vi "test Convert Endpoint to UI Element.vi"(8 "error in (no error)":errorcluster, 11 "TestCase in":refnum<class "SLSC Switch Unit Tests.lvclass">) -> (0 "error out":errorcluster, 3 "TestCase out":refnum<class "SLSC Switch Unit Tests.lvclass">)   [LabVIEW 2017, in "SLSC Switch Unit Tests.lvclass"]
uses:
  SLSC Switch Unit Tests.lvclass
  Shared/Endpoint Configuration Enum.ctl
  System Explorer/Channel Type.ctl
  Shared/Endpoint Configuration Cluster.ctl
  <vilib>/addons/_JKI Toolkits/VI Tester/TestCase.llb/TestCase.lvclass
  System Explorer/SLSC Switch System Explorer.lvlib
  Shared/SLSC Switch Shared.lvlib
  C:/Program Files (x86)/National Instruments/LabVIEW 2017/vi.lib/addons/_JKI Toolkits/VI Tester/TestCase.llb/TestCase.lvclass
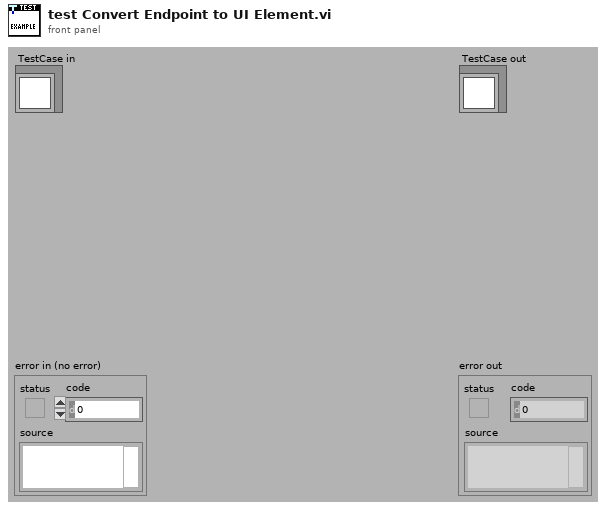
[diagram p1: front panel]
types:
  T1 = typedef "SLSC Switch Shared.lvlib/Endpoint Configuration Enum.ctl" = enum16{"Load", "Source", "Configuration"}
  T2 = typedef "SLSC Switch System Explorer.lvlib/Channel Type.ctl" = enum16{"Load (Default)", "Source", "Configuration"}
  T3 = cluster{"Configuration":T1, "Configuration 2":T2}[]
  T4 = typedef "SLSC Switch Shared.lvlib/Endpoint Configuration Cluster.ctl" = cluster{"Endpoint":string, "Configuration":T1}
  T5 = typedef "SLSC Switch System Explorer.lvlib/Channel.ctl" = cluster{"Endpoint":string, "Configuration":T2}
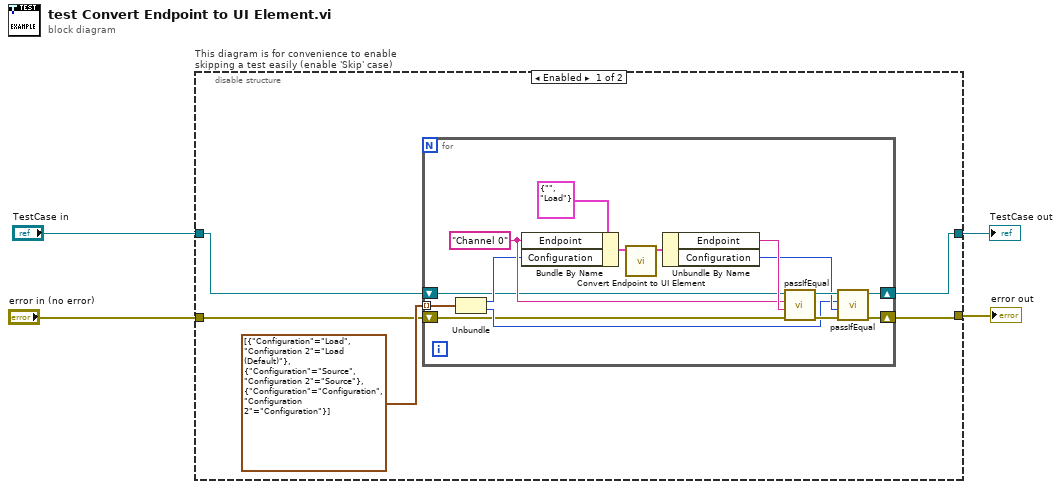
[diagram p0: block diagram]
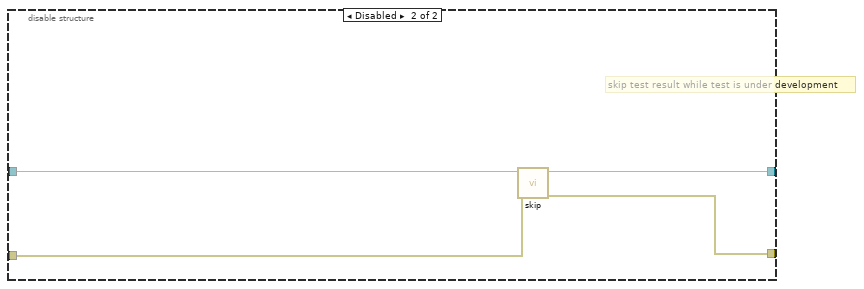
[diagram p2: hidden frame]
diagram:
  n1 = disable-structure "This diagram is for convenience to enable skipping a test easily (enable 'Skip' case)" shown="Enabled" {
    disable-tunnel: "TestCase in" -> [w6 w28]
    disable-tunnel: [w5 w26] -> w1
    disable-tunnel: [w7 w27] -> w3
    disable-tunnel: "error in (no error)" -> [w8 w25]
    frame Enabled {
      n2 = for {
        tunnel: T3 [{"Configuration"=enum."Load", "Configuration 2"=enum."Load (Default)"}, {"Configuration"=enum."Source", "Configuration 2"=enum."Source"}, {"Configuration"=enum."Configuration", "Configuration 2"=enum."Configuration"}] -> [w16] mode=indexing
        shift-right: [w12] -> w7
        shift-left: w8 -> [w13]
        shift-right: [w10] -> w5
        shift-left: w6 -> [w11]
        w18 = "Channel 0" ("Endpoint")
        n3 = Unbundle(w16) -> ("Configuration"=w15:T1, "Configuration 2"=w14:T2)
        n4 = Bundle By Name(cluster=T4 {"Endpoint"="", "Configuration"=enum."Load"} ("Connection"), "Endpoint"=w18, "Configuration"=w15) -> (w22:T4)
        n5 = call "Convert Endpoint to UI Element.vi"("Connection"=w22) -> ("Channel"=w24:T5)  [unwired: 10 in]
        n6 = Unbundle By Name(w24) -> ("Endpoint"=w19:string, "Configuration"=w17:T2)
        n7 = call-dynamic "passIfEqual.vi"("error in (no error)"=w13, "y"=w19, "x"=w18, "TestCase in"=w11) -> ("error out"=w20:errorcluster, "TestCase out"=w21:refnum<class "SLSC Switch Unit Tests.lvclass">)  [unwired: 6 in]
        n8 = call-dynamic "passIfEqual.vi"("error in (no error)"=w20, "y"=w17, "x"=w14, "TestCase in"=w21) -> ("error out"=w12:errorcluster, "TestCase out"=w10:refnum<class "SLSC Switch Unit Tests.lvclass">)  [unwired: 6 in]
      }
    }
    frame Disabled {
      # "skip test result while test is under development"
      n9 = call <vilib>:"skip.vi"("error in (no error)"=w25, "TestCase in"=w28) -> ("error out"=w27:errorcluster, "TestCase out"=w26:refnum<class "SLSC Switch Unit Tests.lvclass">)  [unwired: 8 in]
    }
  }
  "error out" <- w3
  "TestCase out" <- w1
